vi "Config Dialog.vi"(8 "error in (no error)":errorcluster) -> (0 "error out":errorcluster, 2 "Cancelled?":bool, 3 "Configuration File":path)   [LabVIEW 2024]
doc: "Dialog for selecting user specified settings."
uses:
  <vilib>/ErrorRing/Error Ring.xnode
panel:
  in  "Configuration File":path
  in  "Cancel Button":bool
  in  "OK Button":bool
  # "Non visible portion of dialog (needed for connector pane)."
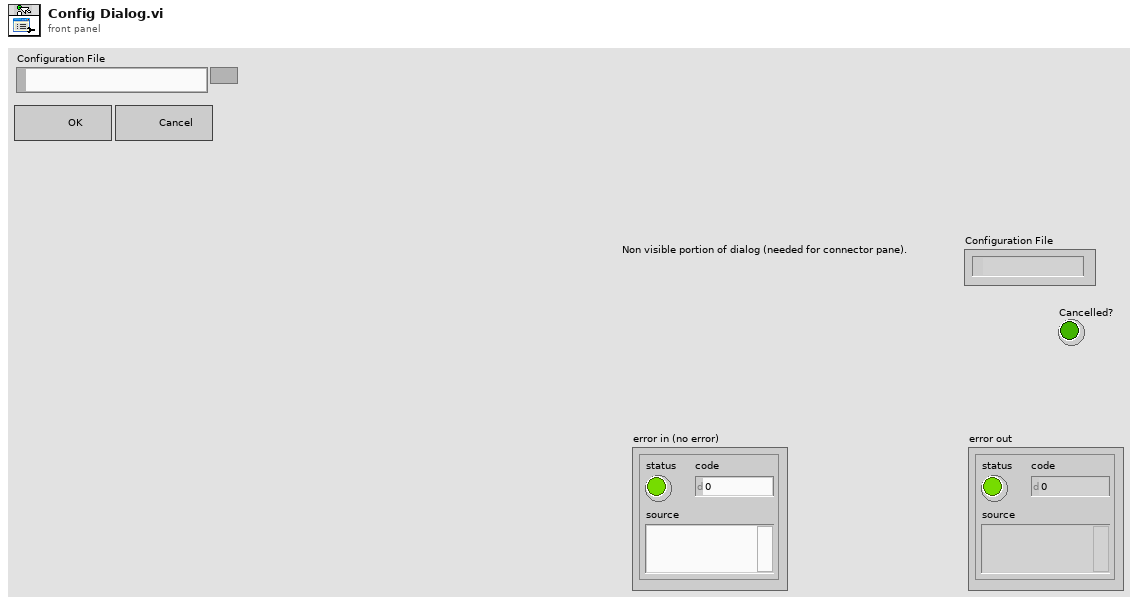
[diagram p1: front panel]
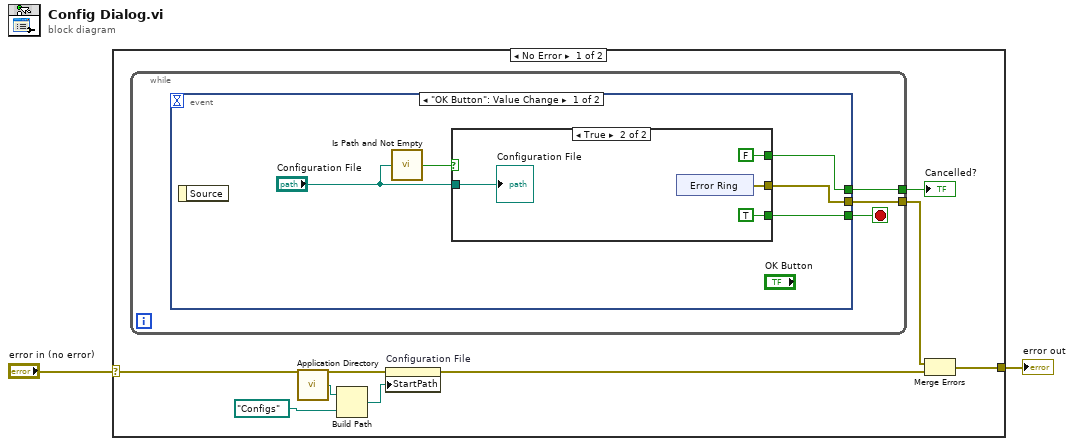
[diagram p0: block diagram]
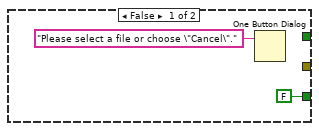
[diagram p2: hidden frame]
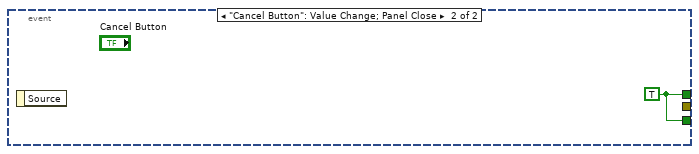
[diagram p3: hidden frame]
diagram:
  n1 = case shown="No Error" "error in (no error)" {
    selector: "error in (no error)" -> [w8 w27]
    tunnel: [w7 w27] -> w2
    frame No Error {
      n2 = while {
        tunnel: [w13] -> w10
        tunnel: [w11] -> w9
        stop <- w12 stop-if-true
        n3 = event shown="[0] \"OK Button\": Value Change" {
          selector: _ -> [_ _]
          dyn-events: _ -> [_ _]
          timeout: _ -> [_ _]
          tunnel: [w18 _] -> w13
          tunnel: [w17 w26] -> w12
          tunnel: [w16 w26] -> w11
          event "OK Button": Value Change {
            n4 = event-data() -> ()  [unwired: 1 in, 1 out]
            n5 = call <vilib>:"Is Path and Not Empty.vi"("path"="Configuration File") -> ("Is Path and Not Empty?"=w15:bool)  [unwired: 4 in]
            n6 = case shown="True" w15 {
              tunnel: "Configuration File" -> [_ w21]
              tunnel: [_ w22] -> w18
              tunnel: [FALSE TRUE] -> w17
              tunnel: [_ FALSE] -> w16
              frame False {
                n7 = One Button Dialog(message="Please select a file or choose \"Cancel\".") -> ()  [unwired: 1 in, 1 out]
              }
              frame True {
                n8 = xnode "Error Ring"() -> ("error out"=w22:errorcluster)
                "Configuration File" <- w21
              }
            }
          }
          event "Cancel Button": Value Change; Panel Close {
            w26 = TRUE
            n9 = event-data() -> ()  [unwired: 1 in, 1 out]
          }
        }
      }
      "Cancelled?" <- w9
      n10 = call <vilib>:"Application Directory.vi"() -> ("Application Directory"=w3:path)
      n11 = Build Path(base path=w3, name or relative path=path "Configs") -> (appended path=w4:path)
      n12 = property on="Configuration File" class="Path"(error in=w8, "StartPath"=w4) -> (error out=w6:errorcluster)  [unwired: 1 in, 1 out]
      n13 = Merge Errors(w10, w6) -> (w7:errorcluster)
    }
    frame Error {
    }
  }
  "error out" <- w2
